vi "Ramp Voltage, New.vi"(0 "offset (0.0)":dbl[unit] format="%.1f", 1 "amplitude (0.0)":dbl[unit] format="%.1f", 2 "dt":dbl[unit]=1e-06 format="%.1f", 3 "total time":dbl[unit]=9.999999999999999e-05 format="%.1f") -> (5 "ramp":dbl[unit][](array[numeric]) format="%.3f")   [LabVIEW 2010]
doc: "This function creates a voltage ramp with respect to time. The first element in the output array will be the offset voltage. If the \"total time\" or dt is zero, then the output ramp will be an empty array."
panel:
  out "dV":dbl[unit]=-1.0
  out "nelem":i32=-1
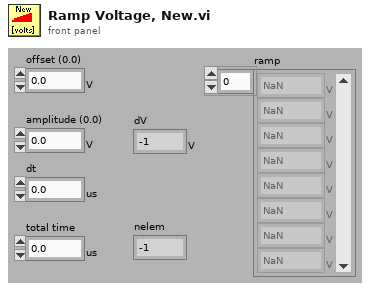
[diagram p1: front panel]
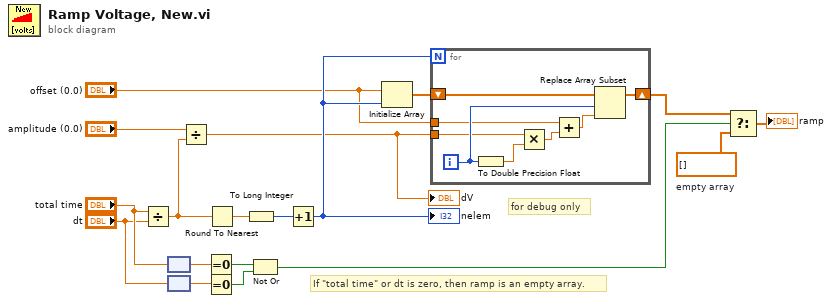
[diagram p0: block diagram]
diagram:
  w1 = dbl[unit][] []  # empty array
  # "If \"total time\" or dt is zero, then ramp is an empty array."
  # "for debug only"
  n1 = Divide(x="total time", y="dt") -> (x/y=w12:dbl)
  n2 = node("total time") -> (w10:dbl)
  n3 = node("dt") -> (w7:dbl)
  n4 = Divide(x="amplitude (0.0)", y=w12) -> (x/y=w11:dbl[unit])
  "dV" <- w11
  n5 = Equal To 0?(x=w10) -> (x = 0?=w6:bool)
  n6 = Equal To 0?(x=w7) -> (x = 0?=w5:bool)
  n7 = Round To Nearest(number=w12) -> (nearest integer value=w17:dbl)
  n8 = To Long Integer(number=w17) -> (32bit integer=w16:i32)
  n9 = Not Or(1:w5, 2:w6) -> (0:w2:bool)
  n10 = Increment(x=w16) -> (x+1=w15:i32)
  "nelem" <- w15
  n11 = Initialize Array("offset (0.0)", w15) -> (w18:dbl[unit][])
  n12 = for {
    N: w15 -> [_]
    shift-right: [w26] -> w4
    shift-left: w18 -> [w25]
    tunnel: w11 -> [w22]
    tunnel: "offset (0.0)" -> [w20]
    i -> [w24]
    n13 = To Double Precision Float(number=w24) -> (double precision float=w23:dbl)
    n14 = Multiply(x=w22, y=w23) -> (x*y=w21:dbl[unit])
    n15 = Add(x=w20, y=w21) -> (x+y=w19:dbl[unit])
    n16 = Replace Array Subset "Replace Array Subset"(array=w25, new element=w19, index=w24) -> (w26:dbl[unit][])
  }
  n17 = Select(t=w4, s=w2, f=w1) -> (s? t:f=→"ramp":dbl[unit][])
